vi "Constants.vi"() -> (4 "VI path":path, 6 "Tests folder name":string="Tests")   [LabVIEW 2016]
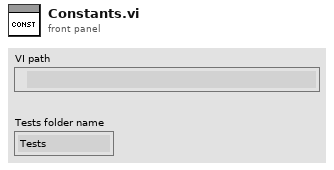
[diagram p1: front panel]
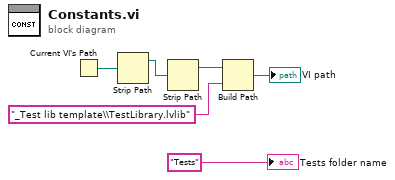
[diagram p0: block diagram]
diagram:
  n1 = Current VI's Path() -> (path=w2:path)
  n2 = Strip Path(path=w2) -> (stripped path=w3:path)  [unwired: 1 out]
  n3 = Strip Path(path=w3) -> (stripped path=w4:path)  [unwired: 1 out]
  n4 = Build Path(base path=w4, name or relative path="_Test lib template\\TestLibrary.lvlib") -> (appended path=→"VI path":path)
  "Tests folder name" <- "Tests" ("name or relative path")
